vi "Install to LVAddons.vi"() -> ()   [LabVIEW 2020]
uses:
  52862042-a624-491b-ba89-58cd6e2a3a21.vi
panel:
  out "error out":errorcluster
  # "NOTE: LabVIEW must be ran in Admin mode for this to work."
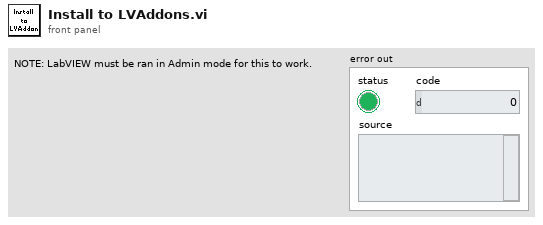
[diagram p1: front panel]
types:
  T1 = enum16{"Create LVAddons folder", "Create lvaddoninfo", "Copy <resource>", "Copy <vi.lib>"}
  T2 = enum16{"Create LVAddons folder", "Create lvaddoninfo", "Copy <resource>", "Copy <vi.lib>"}[]
  T3 = enum16{"open", "replace", "create", "open or create", "replace or create", "replace or create with confirmation"}
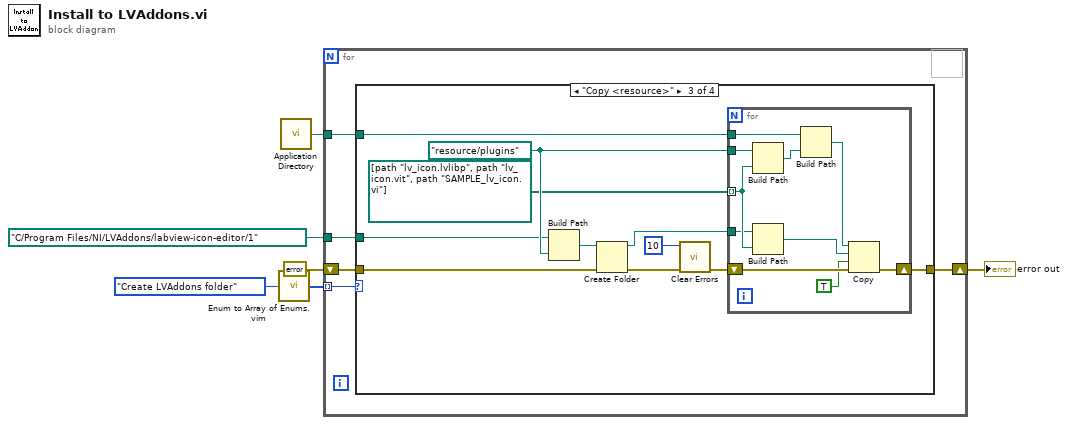
[diagram p0: block diagram]
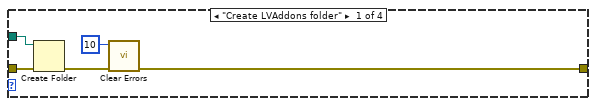
[diagram p2: hidden frame]
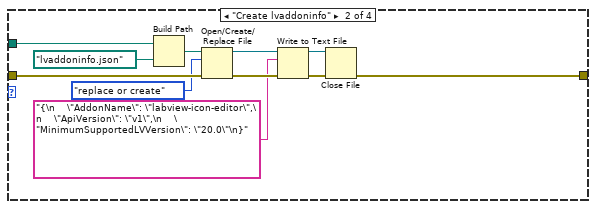
[diagram p3: hidden frame]
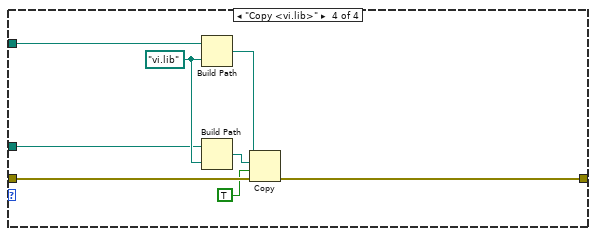
[diagram p4: hidden frame]
diagram:
  n1 = call "Enum to Array of Enums.vim"("enum"=T1."Create LVAddons folder") -> ("array of enums"=w4:T2)
  n2 = call <vilib>:"Application Directory.vi"() -> ("Application Directory"=w1:path)
  n3 = for {
    tunnel: w4 -> [w9] mode=indexing
    tunnel: path "C:/Program Files/NI/LVAddons/labview-icon-editor/1" ("path (use dialog)") -> [w8]
    shift-right: [w11] -> w5
    shift-left: errorcluster {"status"=FALSE, "code"=0, "source"=""} ("error out") -> [w10]
    tunnel: w1 -> [w7]
    n4 = case shown="\"Copy <resource>\"" w9 {
      tunnel: w8 -> [w12 w17 w31 w50]
      tunnel: [w15 w24 w37 w55] -> w11
      tunnel: w10 -> [w14 w25 w38 w56]
      tunnel: w7 -> [_ _ w33 w54]
      frame "Create LVAddons folder" {
        n5 = Create Folder(path (use dialog)=w12, error in=w14) -> (error out=w16:errorcluster)  [unwired: 1 in, 2 out]
        n6 = call <vilib>:"Clear Errors.vi"("error in (no error)"=w16, "specific error code to clear (0: all)"=10) -> ("error out"=w15:errorcluster)  [unwired: 4 in, 1 out]
      }
      frame "Create lvaddoninfo" {
        n7 = Build Path(base path=w17, name or relative path=path "lvaddoninfo.json") -> (appended path=w21:path)
        n8 = Open/Create/Replace File(file path (use dialog)=w21, error in=w25, operation (0:open)=T3."replace or create") -> (refnum out=w22:refnum<file>, error out=w26:errorcluster)  [unwired: 3 in, 1 out]
        n9 = Write to Text File(file (use dialog)=w22, text="{\n    \"AddonName\": \"labview-icon-editor\",\n    \"ApiVersion\": \"v1\",\n    \"MinimumSupportedLVVersion\": \"20.0\"\n}", error in=w26) -> (refnum out=w23:refnum<file>, error out=w27:errorcluster)  [unwired: 1 in, 1 out]
        n10 = Close File(refnum=w23, error in=w27) -> (error out=w24:errorcluster)  [unwired: 1 out]
      }
      frame "Copy <resource>" {
        w34 = path "resource/plugins" ("name or relative path")
        n11 = Build Path(base path=w31, name or relative path=w34) -> (appended path=w30:path)
        n12 = Create Folder(path (use dialog)=w30, error in=w38) -> (created path=w29:path, error out=w36:errorcluster)  [unwired: 1 in, 1 out]
        n13 = call <vilib>:"Clear Errors.vi"("error in (no error)"=w36, "specific error code to clear (0: all)"=10) -> ("error out"=w35:errorcluster)  [unwired: 4 in, 1 out]
        n14 = for {
          shift-right: [w47] -> w37
          shift-left: w35 -> [w48]
          tunnel: w33 -> [w45]
          tunnel: path[] [path "lv_icon.lvlibp", path "lv_icon.vit", path "SAMPLE_lv_icon.vi"] -> [w46] mode=indexing
          tunnel: w34 -> [w43]
          tunnel: w29 -> [w40]
          n15 = Build Path(base path=w43, name or relative path=w46) -> (appended path=w39:path)
          n16 = Build Path(base path=w40, name or relative path=w46) -> (appended path=w42:path)
          n17 = Build Path(base path=w45, name or relative path=w39) -> (appended path=w44:path)
          n18 = Copy(8:w48, 9:TRUE ("overwrite (F)"), 10:w42, 11:w44) -> (0:w47:errorcluster)  [unwired: 1 in, 2 out]
        }
      }
      frame "Copy <vi.lib>" {
        w51 = path "vi.lib" ("name or relative path")
        n19 = Build Path(base path=w54, name or relative path=w51) -> (appended path=w53:path)
        n20 = Build Path(base path=w50, name or relative path=w51) -> (appended path=w49:path)
        n21 = Copy(8:w56, 9:TRUE ("overwrite (F)"), 10:w49, 11:w53) -> (0:w55:errorcluster)  [unwired: 1 in, 2 out]
      }
    }
  }
  "error out" <- w5
